vi "TextControlledInstrumReadCommand.vi"(6 "Operation (read)":T1(ring), 8 "error in (no error)":errorcluster, 9 "timeout in ms (100)":i32=100, 10 "Command":string, 11 "IO Queue":refnum<queue>) -> (0 "error out":errorcluster, 1 "timed out?":bool, 2 "Received":string)   [LabVIEW 2021]
uses:
  TextControlledInstrumIOQueuePacket.ctl
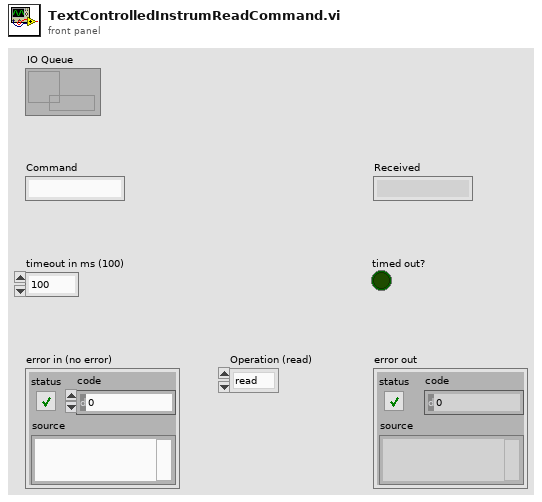
[diagram p1: front panel]
types:
  T1 = enum16{"read", "write", "reserved2", "reserved3", "reserved4", "reserved5", "reserved6", "reserved7"}
  T2 = typedef "TextControlledInstrumIOQueuePacket.ctl" = cluster{"Operation":enum16{"read", "write", "reserved2", "reserved3", "reserved4", "reserved5", "reserved6", "reserved7"}, "Data":string, "Queue":refnum<queue>}
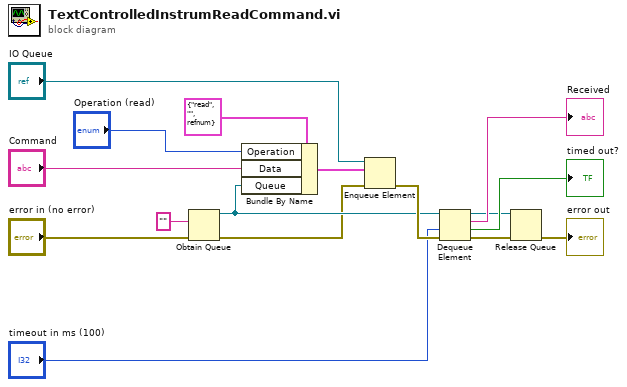
[diagram p0: block diagram]
diagram:
  n1 = Obtain Queue(element data type="", error in (no error)="error in (no error)") -> (queue out=w11:refnum<queue>, error out=w7:errorcluster)  [unwired: 3 in, 1 out]
  n2 = Bundle By Name(cluster=T2 {"Operation"=enum."read", "Data"="", "Queue"=refnum} ("IO Queue Packet"), "Operation"="Operation (read)", "Data"="Command", "Queue"=w11) -> (w15:T2)
  n3 = Enqueue Element(queue="IO Queue", element=w15, error in (no error)=w7) -> (error out=w16:errorcluster)  [unwired: 1 in, 2 out]
  n4 = Dequeue Element(queue=w11, timeout in ms (-1)="timeout in ms (100)", error in (no error)=w16) -> (queue out=w4:refnum<queue>, element=→"Received":string, timed out?=→"timed out?":bool, error out=w2:errorcluster)
  n5 = Release Queue(queue=w4, error in (no error)=w2) -> (error out=→"error out":errorcluster)  [unwired: 1 in, 2 out]
